vi "setup_gui.vi"(0 "Enum":T4(ring), 5 "GUI refnum cluster":T1, 11 "error in (no error)":errorcluster) -> (15 "error out":errorcluster)   [LabVIEW 2013]
uses:
  gui_refnum.ctl
  DDS drivers v3/Array_of_DDS_Boxes.ctl
  DDS drivers v3/DDS_box_cluster.ctl
  DDS drivers v3/DDS_box_device_reference.ctl
  <vilib>/ni845x/ni845x.llb/ni845xControl.ctl
  DDS drivers v3/array_of_DDS_channels.ctl
  DDS drivers v3/DDS_channel.ctl
  DDS drivers v3/array_of_DDS_profiles.ctl
  DDS drivers v3/DDS_profile.ctl
  DDS drivers v3/DDS RAM mode.ctl
  Counter/counter_graph_refnums.ctl
  gui_execution_controls.ctl
  PI_piezo/status.ctl
  <vilib>/vision/Image Controls.llb/IMAQ Image.ctl
  PI_piezo/PI_Piezo.lvclass
  DDS/DDS.lvclass
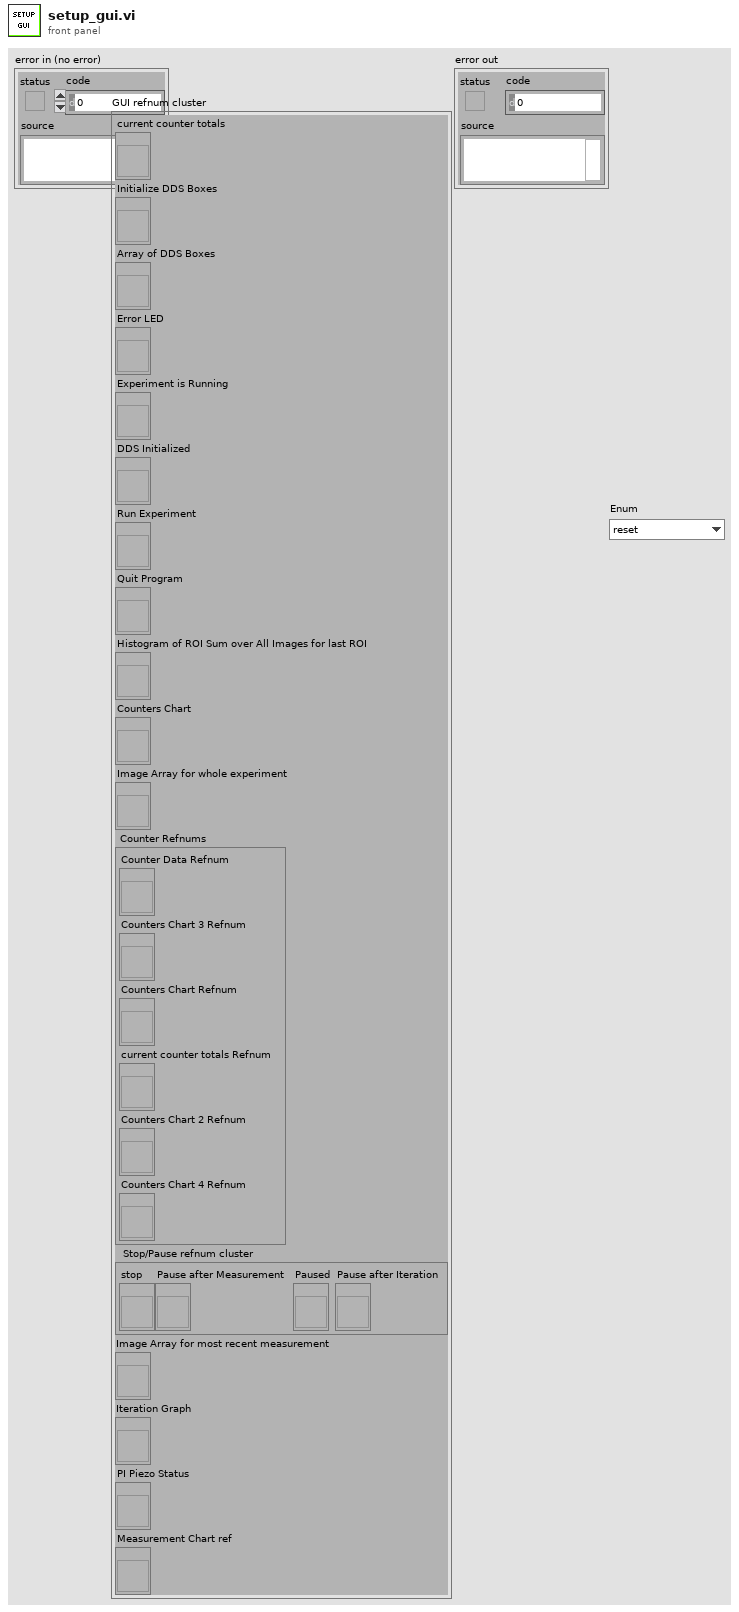
[diagram p1: front panel]
types:
  T1 = typedef "gui_refnum.ctl" = cluster{"current counter totals":refnum<vi>, "Initialize DDS Boxes":refnum<vi>, "Array of DDS Boxes":refnum<vi>, "Error LED":refnum<vi>, "Experiment is Running":refnum<vi>, "DDS Initialized":refnum<vi>, "Run Experiment":refnum<vi>, "Quit Program":refnum<vi>, "Histogram of ROI Sum over All Images for last ROI":refnum<vi>, "Counters Chart":refnum<vi>, "Image Array for whole experiment":refnum<vi>, "Counter Refnums":T2, "Stop/Pause refnum cluster":T3, "Image Array for most recent measurement":refnum<vi>, "Iteration Graph":refnum<vi>, "PI Piezo Status":refnum<vi>, "Measurement Chart ref":refnum<vi>}
  T2 = typedef "counter_graph_refnums.ctl" = cluster{"Counter Data Refnum":refnum<vi>, "Counters Chart 3 Refnum":refnum<vi>, "Counters Chart Refnum":refnum<vi>, "current counter totals Refnum":refnum<vi>, "Counters Chart 2 Refnum":refnum<vi>, "Counters Chart 4 Refnum":refnum<vi>}
  T3 = typedef "gui_execution_controls.ctl" = cluster{"stop":refnum<vi>, "Pause after Measurement":refnum<vi>, "Paused":refnum<vi>, "Pause after Iteration":refnum<vi>}
  T4 = enum16{"reset", "experiment start", "experiment end", "quit"}
  T5 = cluster{"X Values":dbl[], "Histogram: h(x)":i32[]}[]
  T6 = enum8{"Enabled", "Disabled", "Disabled and Grayed Out"}
  T7 = typedef "IMAQ Image.ctl" = refnum<image>
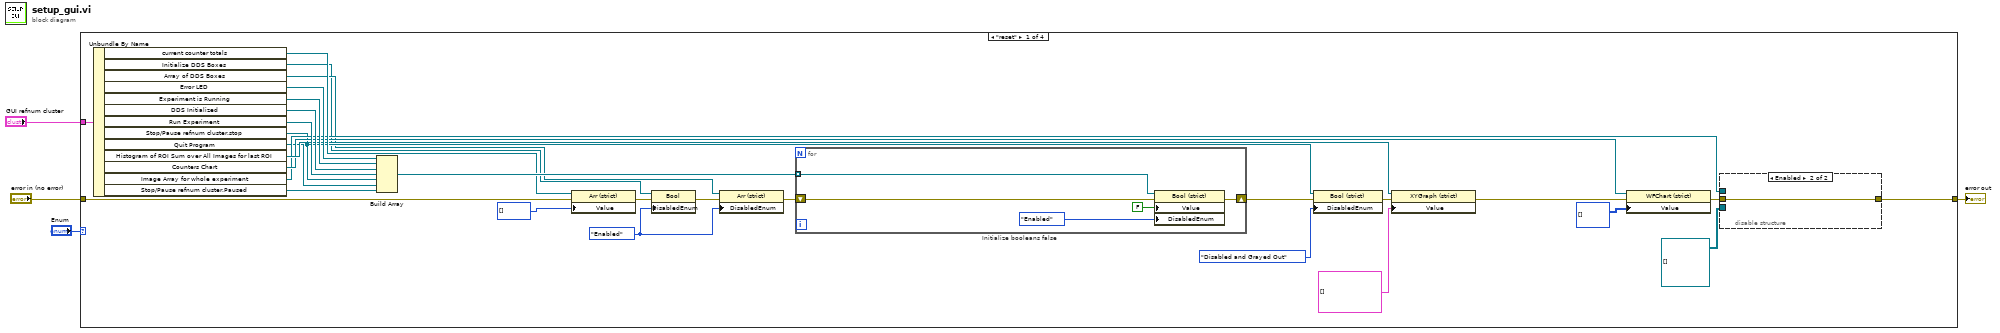
[diagram p0: block diagram]
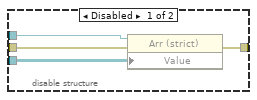
[diagram p2: hidden frame]
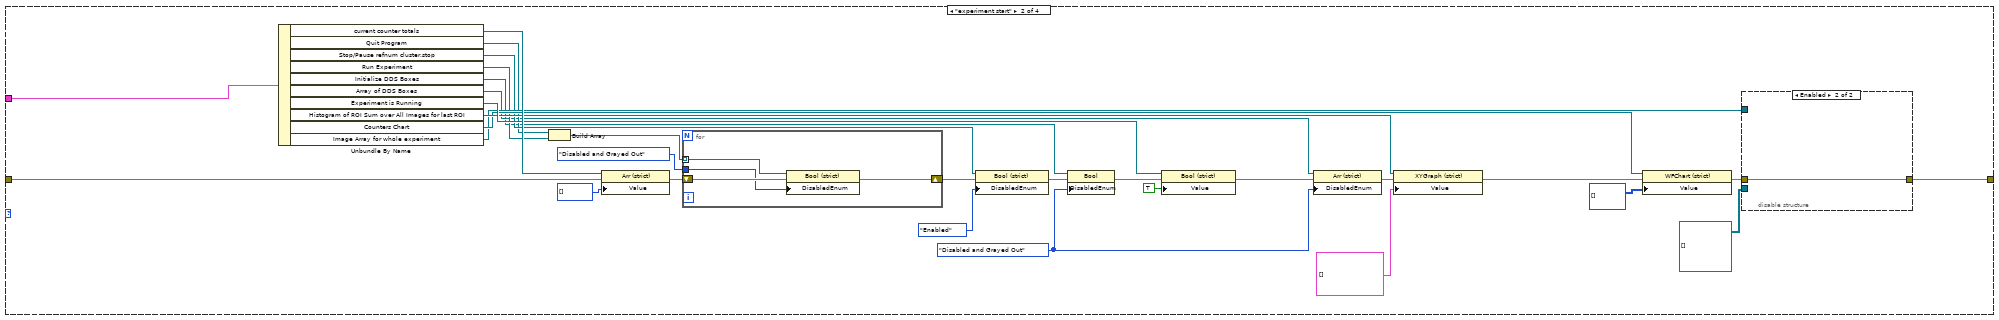
[diagram p3: hidden frame]
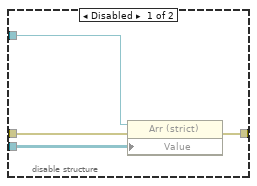
[diagram p4: hidden frame]
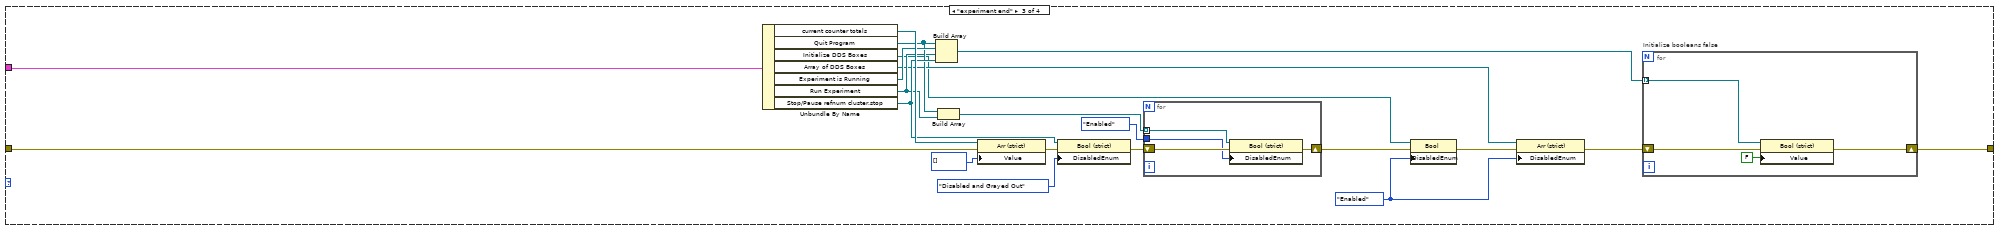
[diagram p5: hidden frame]
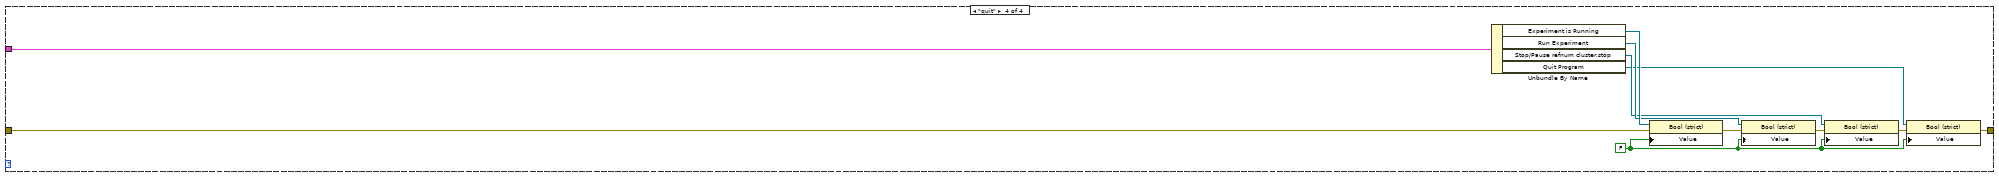
[diagram p6: hidden frame]
diagram:
  n1 = case shown="\"reset\"" "Enum" {
    tunnel: "GUI refnum cluster" -> [w34 w62 w104 w123]
    tunnel: "error in (no error)" -> [w21 w63 w98 w118]
    tunnel: [w16 w64 w95 w113] -> w3
    frame "reset" {
      w14 = T6."Enabled" ("Disabled")
      n2 = Unbundle By Name(w34) -> ("current counter totals"=w28:refnum<vi>, "Initialize DDS Boxes"=w5:refnum<vi>, "Array of DDS Boxes"=w7:refnum<vi>, "Error LED"=w33:refnum<vi>, "Experiment is Running"=w32:refnum<vi>, "DDS Initialized"=w31:refnum<vi>, "Run Experiment"=w30:refnum<vi>, "Stop/Pause refnum cluster.stop"=w11:refnum<vi>, "Quit Program"=w15:refnum<vi>, "Histogram of ROI Sum over All Images for last ROI"=w26:refnum<vi>, "Counters Chart"=w25:refnum<vi>, "Image Array for whole experiment"=w23:refnum<vi>, "Stop/Pause refnum cluster.Paused"=w6:refnum<vi>)
      n3 = Build Array(w33, w32, w31, w30, w11, w15, w6) -> (w29:refnum<vi>[])
      n4 = property class="Arr (strict)"(reference=w28, error in=w21, "Value"=u32[] []) -> (error out=w13:errorcluster)  [unwired: 1 out]
      n5 = property on="Property Node" class="Bool"(reference=w5, error in=w13, "DisabledEnum"=w14) -> (error out=w20:errorcluster)  [unwired: 1 out]
      n6 = property on="Property Node" class="Arr (strict)"(reference=w7, error in=w20, "DisabledEnum"=w14) -> (error out=w19:errorcluster)  [unwired: 1 out]
      n7 = for "Initialize booleans false" {
        tunnel: w29 -> [w43] mode=indexing
        shift-right: [w41] -> w12
        shift-left: w19 -> [w42]
        n8 = property class="Bool (strict)"(reference=w43, error in=w42, "Value"=FALSE, "DisabledEnum"=T6."Enabled" ("Disabled")) -> (error out=w41:errorcluster)  [unwired: 1 out]
      }
      n9 = property class="Bool (strict)"(reference=w11, error in=w12, "DisabledEnum"=T6."Disabled and Grayed Out" ("Disabled")) -> (error out=w10:errorcluster)  [unwired: 1 out]
      n10 = property class="XYGraph (strict)"(reference=w26, error in=w10, "Value"=T5 []) -> (error out=w18:errorcluster)  [unwired: 1 out]
      n11 = property class="WFChart (strict)"(reference=w25, error in=w18, "Value"=u32[][] []) -> (error out=w17:errorcluster)  [unwired: 1 out]
      n12 = disable-structure shown="Enabled" {
        disable-tunnel: w23 -> [w38 _]
        disable-tunnel: T7[][][][] [] ("Value") -> [w37 _]
        disable-tunnel: w17 -> [w36 w39]
        disable-tunnel: [w35 w39] -> w16
        frame Disabled {
          n13 = property class="Arr (strict)"(reference=w38, error in=w36, "Value"=w37) -> (error out=w35:errorcluster)  [unwired: 1 out]
        }
        frame Enabled {
        }
      }
    }
    frame "experiment start" {
      w70 = T6."Disabled and Grayed Out" ("Disabled")
      n14 = Unbundle By Name(w62) -> ("current counter totals"=w61:refnum<vi>, "Quit Program"=w50:refnum<vi>, "Stop/Pause refnum cluster.stop"=w54:refnum<vi>, "Run Experiment"=w49:refnum<vi>, "Initialize DDS Boxes"=w45:refnum<vi>, "Array of DDS Boxes"=w46:refnum<vi>, "Experiment is Running"=w60:refnum<vi>, "Histogram of ROI Sum over All Images for last ROI"=w59:refnum<vi>, "Counters Chart"=w58:refnum<vi>, "Image Array for whole experiment"=w57:refnum<vi>)
      n15 = Build Array(w50, w49) -> (w48:refnum<vi>[])
      n16 = property on="Property Node" class="Arr (strict)"(reference=w61, error in=w63, "Value"=u32[] []) -> (error out=w56:errorcluster)  [unwired: 1 out]
      n17 = for {
        tunnel: w48 -> [w78] mode=indexing
        tunnel: T6."Disabled and Grayed Out" ("Disabled") -> [w76]
        shift-right: [w75] -> w53
        shift-left: w56 -> [w77]
        n18 = property on="Property Node" class="Bool (strict)"(reference=w78, error in=w77, "DisabledEnum"=w76) -> (error out=w75:errorcluster)  [unwired: 1 out]
      }
      n19 = property on="Property Node" class="Bool (strict)"(reference=w54, error in=w53, "DisabledEnum"=T6."Enabled" ("Disabled")) -> (error out=w51:errorcluster)  [unwired: 1 out]
      n20 = property on="Property Node" class="Bool"(reference=w45, error in=w51, "DisabledEnum"=w70) -> (error out=w69:errorcluster)  [unwired: 1 out]
      n21 = property on="Property Node" class="Bool (strict)"(reference=w60, error in=w69, "Value"=TRUE) -> (error out=w68:errorcluster)  [unwired: 1 out]
      n22 = property on="Property Node" class="Arr (strict)"(reference=w46, error in=w68, "DisabledEnum"=w70) -> (error out=w67:errorcluster)  [unwired: 1 out]
      n23 = property on="Property Node" class="XYGraph (strict)"(reference=w59, error in=w67, "Value"=T5 []) -> (error out=w66:errorcluster)  [unwired: 1 out]
      n24 = property on="Property Node" class="WFChart (strict)"(reference=w58, error in=w66, "Value"=u32[][] []) -> (error out=w65:errorcluster)  [unwired: 1 out]
      n25 = disable-structure shown="Enabled" {
        disable-tunnel: w57 -> [w82 _]
        disable-tunnel: T7[][][][] [] ("Value") -> [w81 _]
        disable-tunnel: w65 -> [w80 w83]
        disable-tunnel: [w79 w83] -> w64
        frame Disabled {
          n26 = property on="Property Node" class="Arr (strict)"(reference=w82, error in=w80, "Value"=w81) -> (error out=w79:errorcluster)  [unwired: 1 out]
        }
        frame Enabled {
        }
      }
    }
    frame "experiment end" {
      w101 = T6."Enabled" ("Disabled")
      n27 = Unbundle By Name(w104) -> ("current counter totals"=w103:refnum<vi>, "Quit Program"=w89:refnum<vi>, "Initialize DDS Boxes"=w84:refnum<vi>, "Array of DDS Boxes"=w85:refnum<vi>, "Experiment is Running"=w100:refnum<vi>, "Run Experiment"=w86:refnum<vi>, "Stop/Pause refnum cluster.stop"=w94:refnum<vi>)
      n28 = Build Array(w89, w100, w86, w94) -> (w99:refnum<vi>[])
      n29 = Build Array(w89, w86) -> (w91:refnum<vi>[])
      n30 = property on="Property Node" class="Arr (strict)"(reference=w103, error in=w98, "Value"=u32[] []) -> (error out=w93:errorcluster)  [unwired: 1 out]
      n31 = property on="Property Node" class="Bool (strict)"(reference=w94, error in=w93, "DisabledEnum"=T6."Disabled and Grayed Out" ("Disabled")) -> (error out=w88:errorcluster)  [unwired: 1 out]
      n32 = for {
        tunnel: w91 -> [w108] mode=indexing
        tunnel: T6."Enabled" ("Disabled") -> [w106]
        shift-right: [w105] -> w87
        shift-left: w88 -> [w107]
        n33 = property on="Property Node" class="Bool (strict)"(reference=w108, error in=w107, "DisabledEnum"=w106) -> (error out=w105:errorcluster)  [unwired: 1 out]
      }
      n34 = property on="Property Node" class="Bool"(reference=w84, error in=w87, "DisabledEnum"=w101) -> (error out=w97:errorcluster)  [unwired: 1 out]
      n35 = property on="Property Node" class="Arr (strict)"(reference=w85, error in=w97, "DisabledEnum"=w101) -> (error out=w96:errorcluster)  [unwired: 1 out]
      n36 = for "Initialize booleans false" {
        tunnel: w99 -> [w111] mode=indexing
        shift-right: [w109] -> w95
        shift-left: w96 -> [w110]
        n37 = property class="Bool (strict)"(reference=w111, error in=w110, "Value"=FALSE) -> (error out=w109:errorcluster)  [unwired: 1 out]
      }
    }
    frame "quit" {
      w114 = FALSE ("Value")
      n38 = Unbundle By Name(w123) -> ("Experiment is Running"=w122:refnum<vi>, "Run Experiment"=w121:refnum<vi>, "Stop/Pause refnum cluster.stop"=w120:refnum<vi>, "Quit Program"=w119:refnum<vi>)
      n39 = property class="Bool (strict)"(reference=w122, error in=w118, "Value"=w114) -> (error out=w117:errorcluster)  [unwired: 1 out]
      n40 = property class="Bool (strict)"(reference=w121, error in=w117, "Value"=w114) -> (error out=w116:errorcluster)  [unwired: 1 out]
      n41 = property class="Bool (strict)"(reference=w120, error in=w116, "Value"=w114) -> (error out=w115:errorcluster)  [unwired: 1 out]
      n42 = property class="Bool (strict)"(reference=w119, error in=w115, "Value"=w114) -> (error out=w113:errorcluster)  [unwired: 1 out]
    }
  }
  "error out" <- w3
